vi "Create Canonicalized Resource.vi"(10 "HTTP Session in":refnum<class "Session.lvclass">) -> (2 "Canonical resource":string, 3 "HTTP Session out":refnum<class "Session.lvclass">)   [LabVIEW 2015, in "NI_Azure_Core.lvlib" / "Session.lvclass"]
uses:
  Session.lvclass
  <vilib>/Utility/error.llb/whitespace.ctl
  Format Request Parameters Mode.ctl
  Session.lvclass/Session.ctl
  Read URL Suffix.vi
  Read Request Parameters.vi
  Read Storage Account Name.vi
  NI_Azure_Core.lvlib
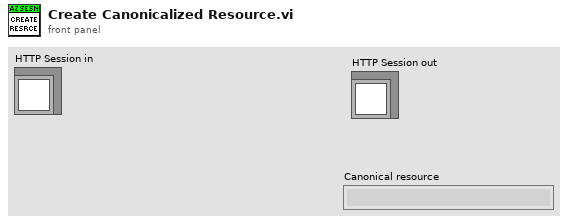
[diagram p1: front panel]
types:
  T1 = typedef "NI_Azure_Core.lvlib/Format Request Parameters Mode.ctl" = enum16{"URL", "Signing"}
  T2 = typedef "whitespace.ctl" = u16
  T3 = typedef "NI_Azure_Core.lvlib/Name Value Pair.ctl" = cluster{"name":string, "value":string}
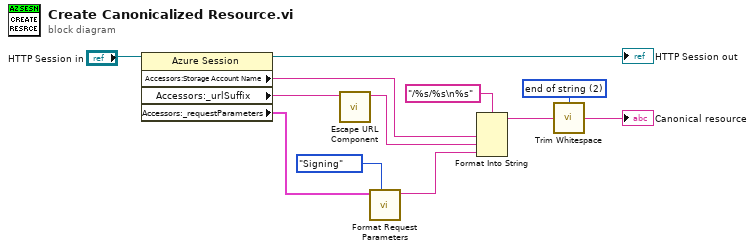
[diagram p0: block diagram]
diagram:
  w9 = T2 2 items=["both", "start of string", "end of string"] ("location (both)")
  n1 = property class="Azure Session"(reference="HTTP Session in") -> (reference out=→"HTTP Session out":refnum<class "Session.lvclass">, "Accessors:Storage Account Name"=w3:string, "Accessors:_urlSuffix"=w2:string, "Accessors:_requestParameters"=w5:T3[])  [unwired: 1 in, 1 out]
  n2 = call "Escape URL Component.vi"("URL component in"=w2) -> ("URL component out"=w1:string)  [unwired: 10 in]
  n3 = call "Format Request Parameters.vi"("Mode"=Format_Request_Parameters_Mode."Signing", "Request parameters"=w5) -> ("Parameter string"=w4:string)  [unwired: 9 in]
  n4 = Format Into String(format string="/%s/%s\n%s" ("string"), w3, w1, w4) -> (resulting string=w7:string)  [unwired: 2 in, 1 out]
  n5 = call <vilib>:"Trim Whitespace.vi"("string"=w7, "location (both)"=w9) -> ("trimmed string"=→"Canonical resource":string)
